vi "Calculate Sample Buffer Size.vi"(10 "Reverse (F)":bool, 11 "Speed Multiplier":dbl format="%#_13g") -> (3 "Sample Size":i32)   [LabVIEW 2019, in "Audio Processing.lvlib"]
doc: "Calculate the size of the audio buffer based on the playback speed."
uses:
  Audio Processing.lvlib
  Globals/Constants.vi
  Globals/Globals.lvlib
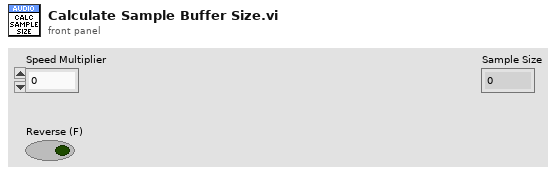
[diagram p1: front panel]
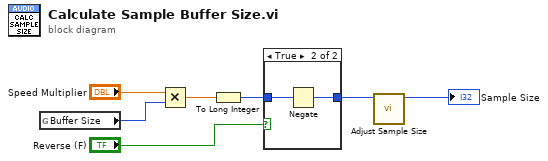
[diagram p0: block diagram]
diagram:
  n1 = global read "Constants.vi" "Buffer Size"() -> (w4:i32)
  n2 = Multiply(x="Speed Multiplier", y=w4) -> (x*y=w3:dbl)
  n3 = To Long Integer(number=w3) -> (32bit integer=w2:i32)
  n4 = case shown="True" "Reverse (F)" {
    tunnel: w2 -> [w8 w10]
    tunnel: [w8 w9] -> w1
    frame False {
    }
    frame True {
      n5 = Negate(x=w10) -> (-x=w9:i32)
    }
  }
  n6 = call "Adjust Sample Size.vi"("Sample Size In"=w1) -> ("Sample Size Out"=→"Sample Size":i32)  [unwired: 10 in]
